vi "Husky Loop.vi"() -> ()   [LabVIEW 2011]
uses:
  clearpath_interface.lvlib
panel:
  in  "Set Velocity 2":bool
  in  "Translational Speed 2":dbl
  in  "Rotational Speed 2":dbl
  in  "Set Brake 2":bool
  in  "Continuous Vel 2":bool
  in  "Debug":bool
  in  "VISA resource name":refnum<visa-resource-name>
  out "Charge":dbl(slide) scale=0.0..100.0
  out "Left Speed (m/s)":dbl
  out "Right Speed (m/s)":dbl
  out "Capacity":i16
  out "Flags":u8 format="%b"
  out "Flags 2":u8 format="%x"
  in  "End Loop":bool
  in  "stop?":bool
  in  "Reset":bool
  in  "Max Accel":dbl
  in  "Set Max Accel":bool
  in  "Max Speed":dbl
  in  "Set Max Speed":bool
  in  "Set Velocity":bool
  in  "Translational Speed":dbl
  in  "Rotational Speed":dbl
  in  "Set Brake":bool
  in  "Continuous Vel":bool
  in  "Right Output":dbl
  in  "Left Output":dbl
  in  "Continuous Output":bool
  in  "Set Output":bool
  in  "P":dbl
  in  "I":dbl
  in  "D":dbl
  in  "FF":dbl
  in  "Stic":dbl
  in  "Int Lim":dbl
  in  "Set Controls":bool
  in  "Right Speed":dbl
  in  "Left Speed":dbl
  in  "Left Accel":dbl
  in  "Right Accel":dbl
  in  "Continuous Speeds":bool
  in  "Set Speeds":bool
  in  "Remote E-Stop":bool
  in  "Set Safety":bool
  in  "New Chassis Time (ms)":u32
  in  "Set Time":bool
  in  "New Chassis Name":string
  in  "Set Name":bool
  in  "FreqRawEncoder":u8
  in  "Update Raw Encoders":bool
  in  "Update Encoder":bool
  in  "FreqEncoder":u8
  in  "FreqPlatformRot":u8
  in  "Update Platform Rotation":bool
  in  "FreqMaxAccel":u8
  in  "Update Max Accel":bool
  in  "FreqMaxSpeed":u8
  in  "Update Max Speed":bool
  in  "FreqDifferentialOutput":u8
  in  "Update Differential Output":bool
  in  "FreqDifferentialControl":u8
  in  "Update Differential Control":bool
  in  "FreqDifferentialSpeed":u8
  in  "Update Differential Speed":bool
  in  "FreqSafetyStatus":u8
  in  "Update Safety Status":bool
  in  "FreqPowerSystem":u8
  in  "Update Power System":bool
  in  "FreqSystemStatus":u8
  in  "Update System Status":bool
  in  "FreqFirmwareInfo":u8
  in  "Update Firmware Info":bool
  in  "FreqPlatformName":u8
  in  "Update Platform Name":bool
  in  "FreqPlatformInfo":u8
  in  "Update Platform Info":bool
  # "Subscriptions"
  # "Communication Status"
  # "Platform Info (0x8001)"
  # "Differential Control (0x8201)"
  # "Platform Name (0x8002)"
  # "Differential Output (0x8202)"
  # "Firmware Info (0x8003)"
  # "Max Speed (0x8210)"
  # "System Status (0x8004)"
  # "Max Accel (0x8211)"
  # "Power System (0x8005)"
  # "Platform Rotation (0x8601)"
  # "Safety System Status (0x8010)"
  # "Encoders (0x8800)"
  # "Differential Speed (0x8200)"
  # "Raw Encoders (0x8801)"
  # "Set Velocity"
  # "Set Differential Speeds"
  # "Set Chassis Name/Time"
  # "Set Differential Controls"
  # "Set Differential Output"
  # "Set Max Speed/Accel"
  # "Set Safety System"
  # "Reset Processor"
  # "Control Test Panel\nClearpath Control Protocol cRIO Test Interface v1.0\nClearpath Robotics Inc., (c) 2010"
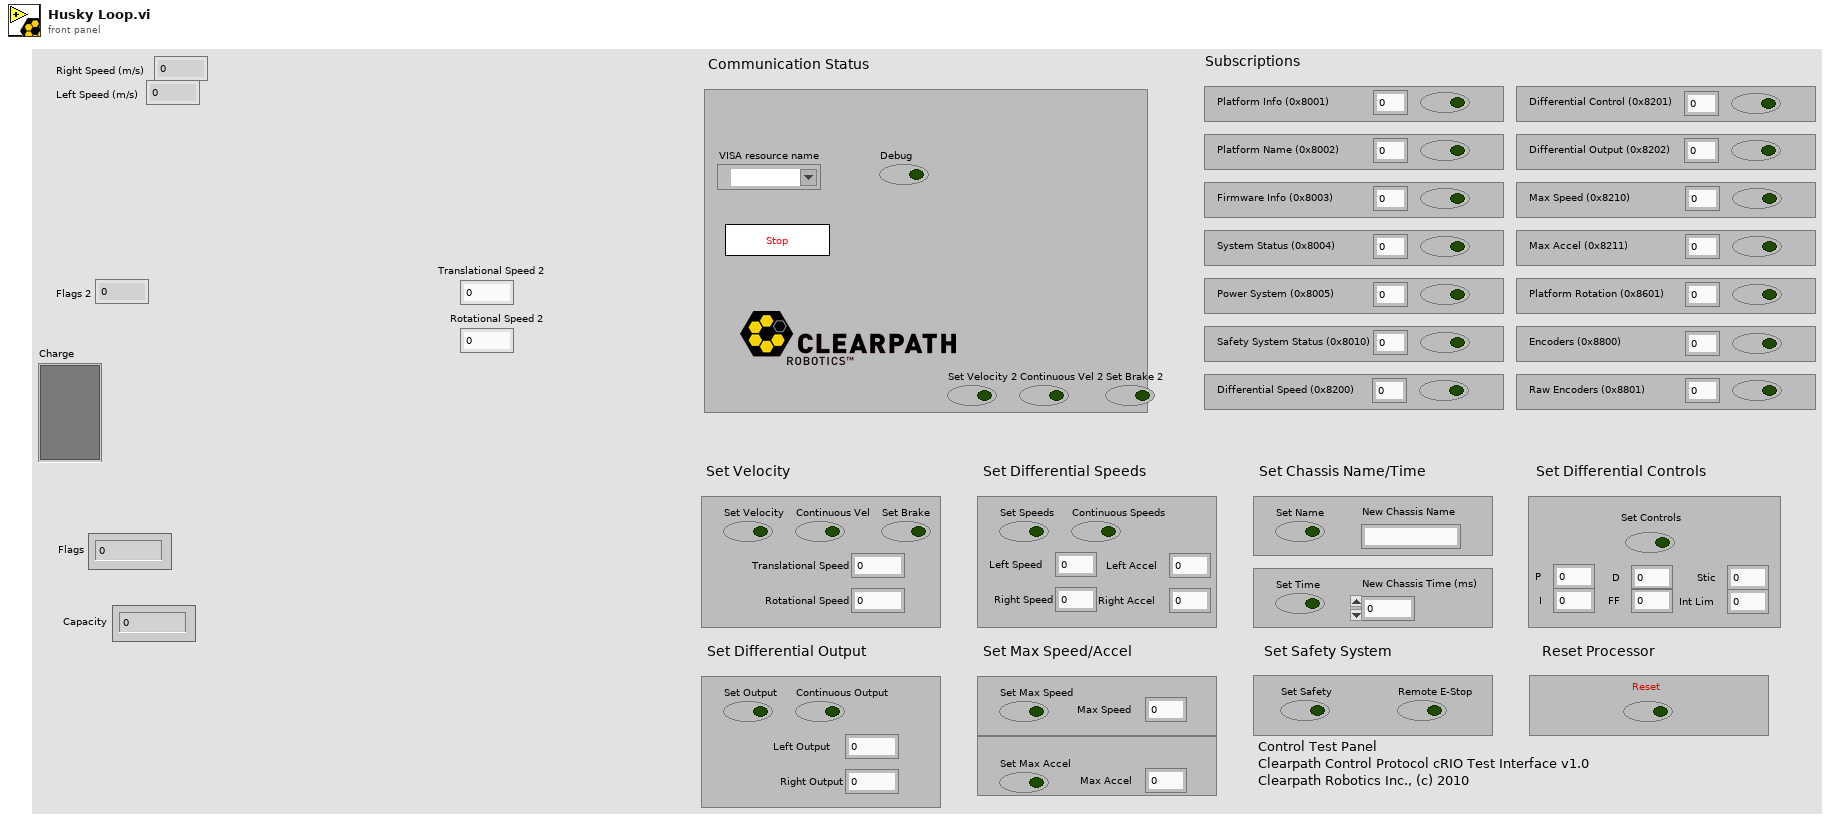
[diagram p1: front panel]
types:
  T1 = cluster{"P":dbl, "I":dbl, "D":dbl, "FF":dbl, "Stic":dbl, "Int Lim":dbl}
  T2 = cluster{"Xmit Queue":refnum<queue>, "Data Queue":refnum<queue>, "VISA resource name out":refnum<visa-resource-name>, "error out":errorcluster, "Message Data Cluster":cluster{"\nChar Idx":u8, "Num. Char Rem":u8, "Write Index":u8, "Read Index":u8, "Message Data Buffer":u8[][]}}
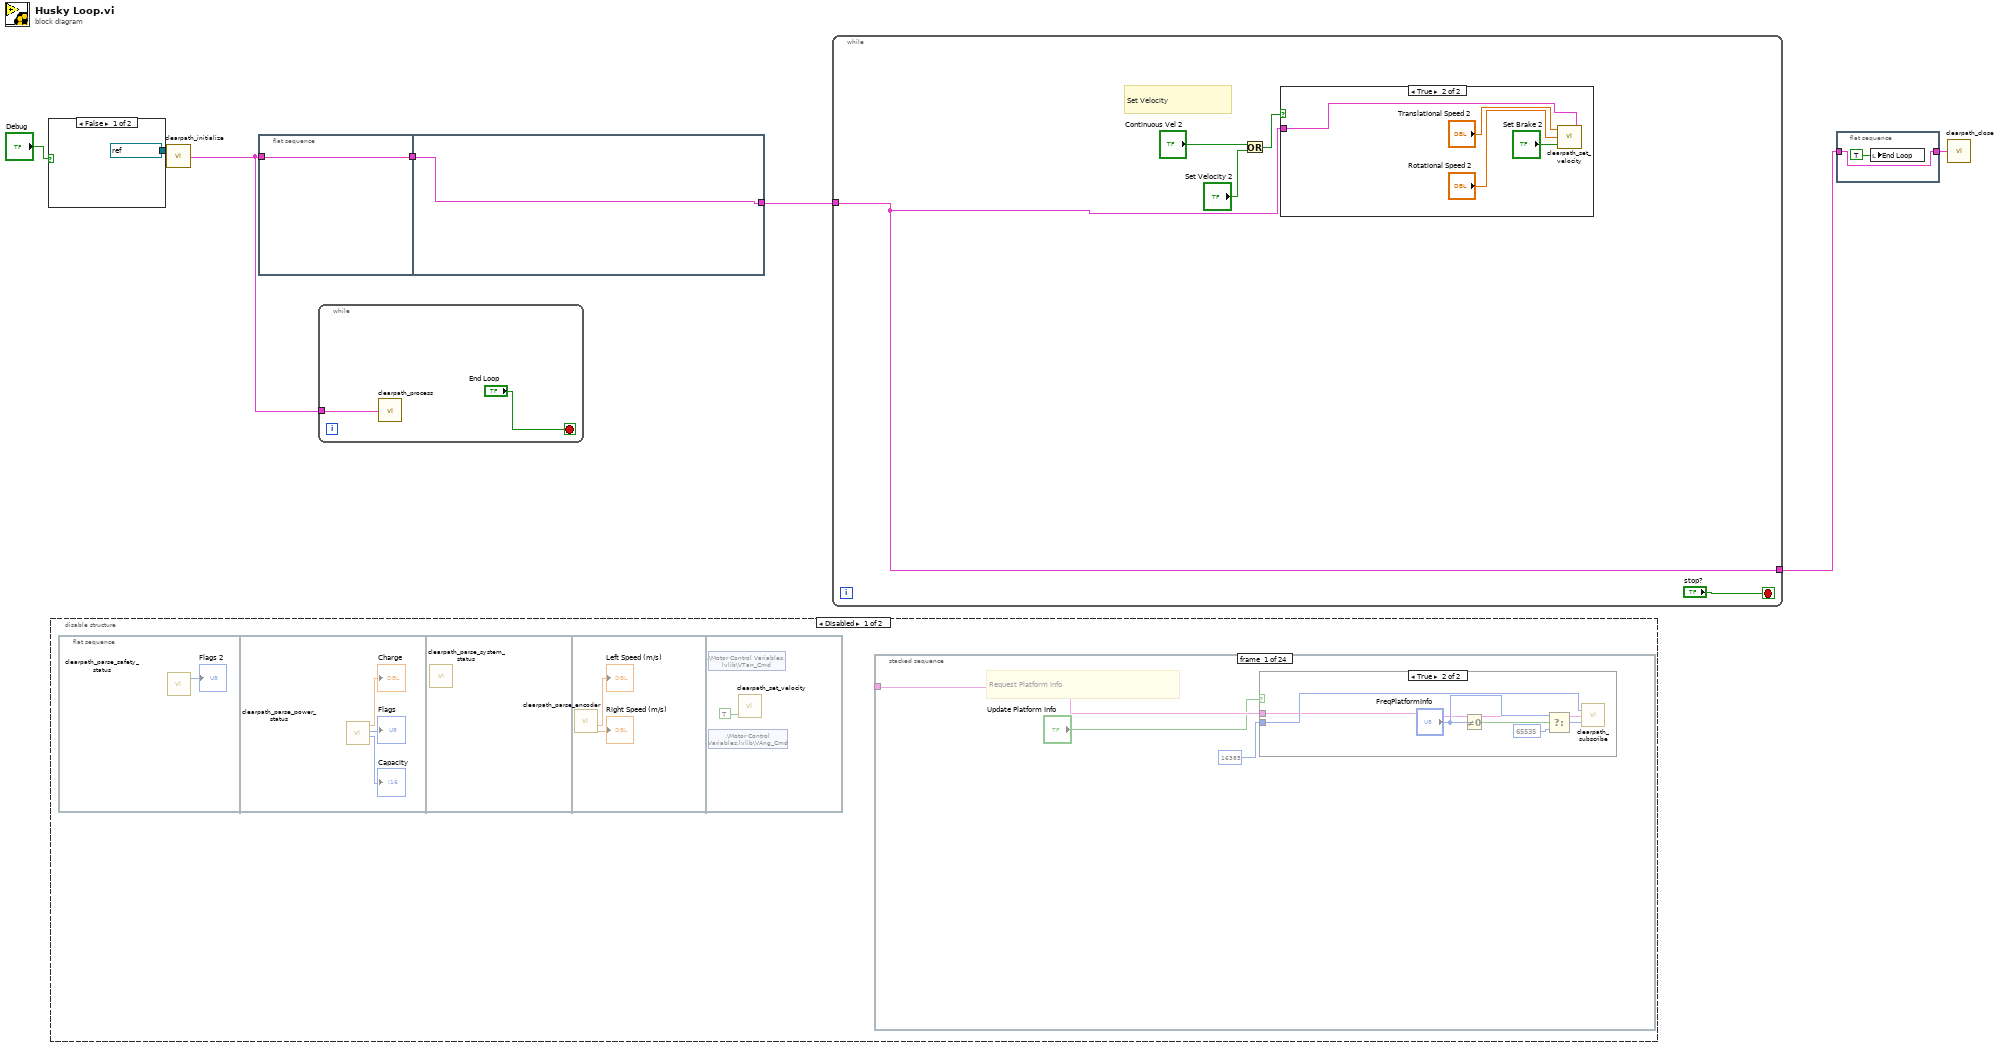
[diagram p0: block diagram]
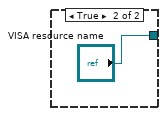
[diagram p3: hidden frame]
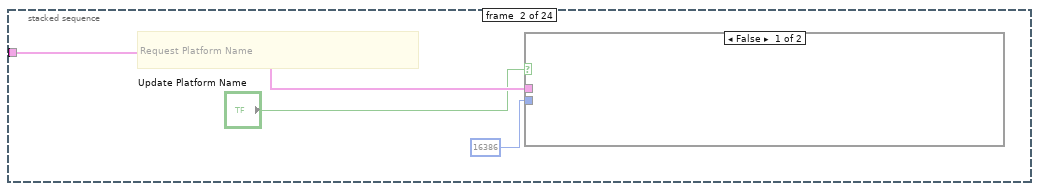
[diagram p5: hidden frame]
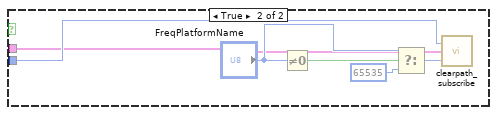
[diagram p6: hidden frame]
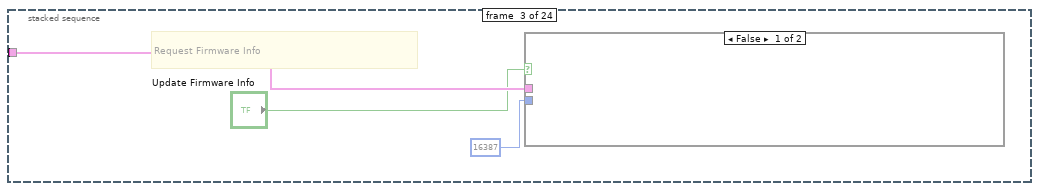
[diagram p7: hidden frame]
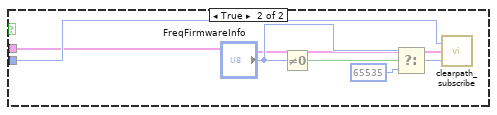
[diagram p8: hidden frame]
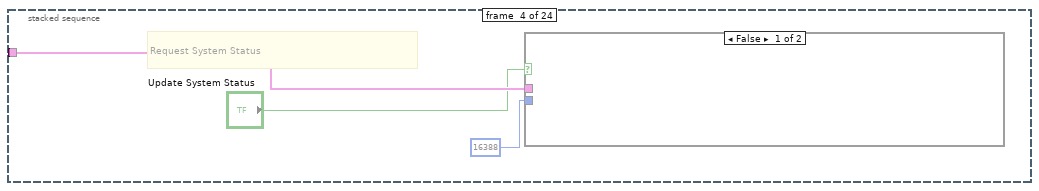
[diagram p9: hidden frame]
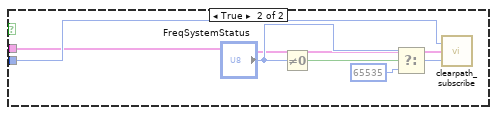
[diagram p10: hidden frame]
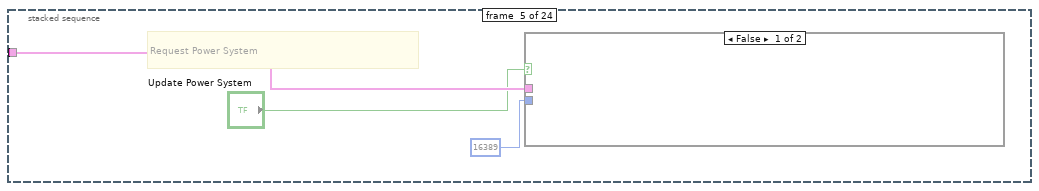
[diagram p11: hidden frame]
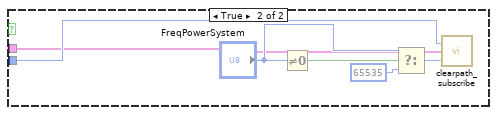
[diagram p12: hidden frame]
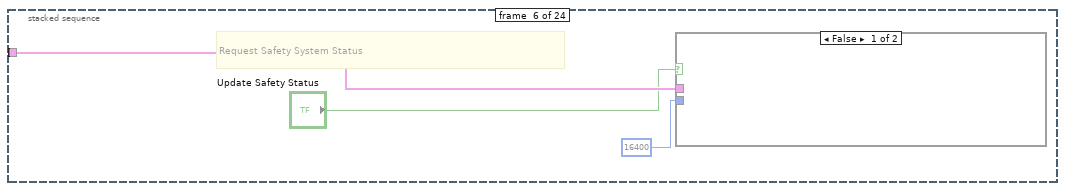
[diagram p13: hidden frame]
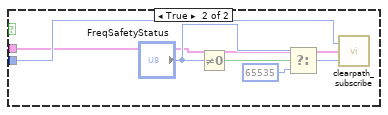
[diagram p14: hidden frame]
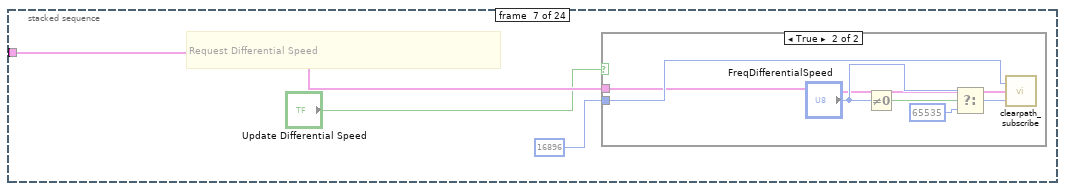
[diagram p15: hidden frame]
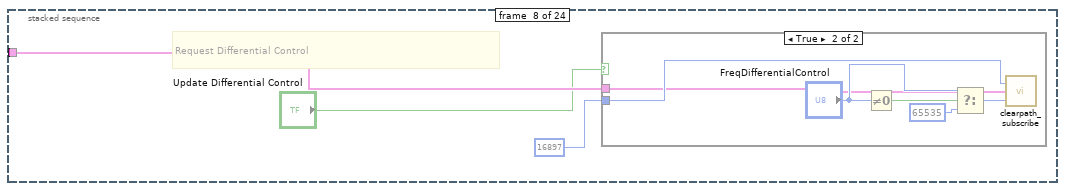
[diagram p17: hidden frame]
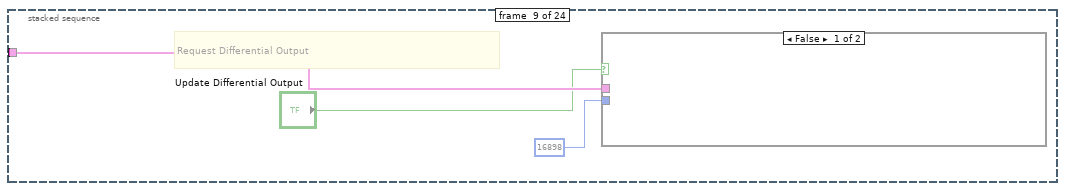
[diagram p19: hidden frame]
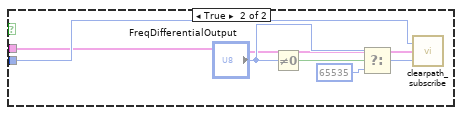
[diagram p20: hidden frame]
diagram:
  n1 = case shown="False" "Debug" {
    tunnel: [refnum<visa-resource-name> "COM15" ("VISA resource name") "VISA resource name"] -> w7
    frame False {
    }
    frame True {
    }
  }
  n2 = disable-structure shown="Disabled" {
    frame Disabled {
      n3 = flat-sequence {
        frame #0 {
          n4 = call "clearpath_parse_safety_status.vi"() -> ("Flags"=→"Flags 2":u8)  [unwired: 1 in, 1 out]
        }
        frame #1 {
          n5 = call "clearpath_parse_power_status.vi"() -> ("Capacity"=→"Capacity":i16, "Flags"=→"Flags":u8, "Charge"=→"Charge":dbl)  [unwired: 1 in, 1 out]
        }
        frame #2 {
          n6 = call "clearpath_parse_system_status.vi"() -> ()  [unwired: 1 in, 6 out]
        }
        frame #3 {
          n7 = call "clearpath_parse_encoder.vi"() -> ("Left Speed (m/s)"=→"Left Speed (m/s)":dbl, "Right Speed (m/s)"=→"Right Speed (m/s)":dbl)  [unwired: 1 in, 3 out]
        }
        frame #4 {
          n8 = shared-variable ".\\Motor Control Variables.lvlib\\VTan_Cmd"() -> ()  [unwired: 1 in, 2 out]
          n9 = shared-variable ".\\Motor Control Variables.lvlib\\VAng_Cmd"() -> ()  [unwired: 1 in, 2 out]
          n10 = call "clearpath_set_velocity.vi"("Zero Speeds"=TRUE) -> ()  [unwired: 3 in]
        }
      }
      n11 = stacked-sequence {
        tunnel: _ -> [w11 w21 w29 w38 w47 w56 w65 w74 w83 w92 w101 w111 w120 w129 w137 w141 w145 w150 w157 w168 w174 w181 w185 w189]
        frame #0 {
          # "Request Platform Info"
          n12 = case shown="True" "Update Platform Info" {
            tunnel: w11 -> [_ w13]
            tunnel: 16385 -> [_ w18]
            frame False {
            }
            frame True {
              n13 = Not Equal To 0?(x="FreqPlatformInfo") -> (x != 0?=w16:bool)
              n14 = Select(t="FreqPlatformInfo", s=w16, f=u16 65535) -> (s? t:f=w15:u16)
              n15 = call "clearpath_subscribe.vi"("ClearpathComm"=w13, "Frequency"=w15, "Message Type"=w18) -> ()
            }
          }
        }
        frame #1 {
          # "Request Platform Name"
          n16 = case shown="False" "Update Platform Name" {
            tunnel: w21 -> [_ w22]
            tunnel: 16386 -> [_ w27]
            frame False {
            }
            frame True {
              n17 = Not Equal To 0?(x="FreqPlatformName") -> (x != 0?=w25:bool)
              n18 = Select(t="FreqPlatformName", s=w25, f=u16 65535) -> (s? t:f=w24:u16)
              n19 = call "clearpath_subscribe.vi"("ClearpathComm"=w22, "Frequency"=w24, "Message Type"=w27) -> ()
            }
          }
        }
        frame #2 {
          # "Request Firmware Info"
          n20 = case shown="False" "Update Firmware Info" {
            tunnel: w29 -> [_ w31]
            tunnel: 16387 -> [_ w36]
            frame False {
            }
            frame True {
              n21 = Not Equal To 0?(x="FreqFirmwareInfo") -> (x != 0?=w34:bool)
              n22 = Select(t="FreqFirmwareInfo", s=w34, f=u16 65535) -> (s? t:f=w33:u16)
              n23 = call "clearpath_subscribe.vi"("ClearpathComm"=w31, "Frequency"=w33, "Message Type"=w36) -> ()
            }
          }
        }
        frame #3 {
          # "Request System Status"
          n24 = case shown="False" "Update System Status" {
            tunnel: w38 -> [_ w40]
            tunnel: 16388 -> [_ w45]
            frame False {
            }
            frame True {
              n25 = Not Equal To 0?(x="FreqSystemStatus") -> (x != 0?=w43:bool)
              n26 = Select(t="FreqSystemStatus", s=w43, f=u16 65535) -> (s? t:f=w42:u16)
              n27 = call "clearpath_subscribe.vi"("ClearpathComm"=w40, "Frequency"=w42, "Message Type"=w45) -> ()
            }
          }
        }
        frame #4 {
          # "Request Power System"
          n28 = case shown="False" "Update Power System" {
            tunnel: w47 -> [_ w49]
            tunnel: 16389 -> [_ w54]
            frame False {
            }
            frame True {
              n29 = Not Equal To 0?(x="FreqPowerSystem") -> (x != 0?=w52:bool)
              n30 = Select(t="FreqPowerSystem", s=w52, f=u16 65535) -> (s? t:f=w51:u16)
              n31 = call "clearpath_subscribe.vi"("ClearpathComm"=w49, "Frequency"=w51, "Message Type"=w54) -> ()
            }
          }
        }
        frame #5 {
          # "Request Safety System Status"
          n32 = case shown="False" "Update Safety Status" {
            tunnel: w56 -> [_ w58]
            tunnel: 16400 -> [_ w63]
            frame False {
            }
            frame True {
              n33 = Not Equal To 0?(x="FreqSafetyStatus") -> (x != 0?=w61:bool)
              n34 = Select(t="FreqSafetyStatus", s=w61, f=u16 65535) -> (s? t:f=w60:u16)
              n35 = call "clearpath_subscribe.vi"("ClearpathComm"=w58, "Frequency"=w60, "Message Type"=w63) -> ()
            }
          }
        }
        frame #6 {
          # "Request Differential Speed"
          n36 = case shown="True" "Update Differential Speed" {
            tunnel: w65 -> [_ w67]
            tunnel: 16896 -> [_ w72]
            frame False {
            }
            frame True {
              n37 = Not Equal To 0?(x="FreqDifferentialSpeed") -> (x != 0?=w70:bool)
              n38 = Select(t="FreqDifferentialSpeed", s=w70, f=u16 65535) -> (s? t:f=w69:u16)
              n39 = call "clearpath_subscribe.vi"("ClearpathComm"=w67, "Frequency"=w69, "Message Type"=w72) -> ()
            }
          }
        }
        frame #7 {
          # "Request Differential Control"
          n40 = case shown="True" "Update Differential Control" {
            tunnel: w74 -> [_ w76]
            tunnel: 16897 -> [_ w81]
            frame False {
            }
            frame True {
              n41 = Not Equal To 0?(x="FreqDifferentialControl") -> (x != 0?=w79:bool)
              n42 = Select(t="FreqDifferentialControl", s=w79, f=u16 65535) -> (s? t:f=w78:u16)
              n43 = call "clearpath_subscribe.vi"("ClearpathComm"=w76, "Frequency"=w78, "Message Type"=w81) -> ()
            }
          }
        }
        frame #8 {
          # "Request Differential Output"
          n44 = case shown="False" "Update Differential Output" {
            tunnel: w83 -> [_ w85]
            tunnel: 16898 -> [_ w90]
            frame False {
            }
            frame True {
              n45 = Not Equal To 0?(x="FreqDifferentialOutput") -> (x != 0?=w88:bool)
              n46 = Select(t="FreqDifferentialOutput", s=w88, f=u16 65535) -> (s? t:f=w87:u16)
              n47 = call "clearpath_subscribe.vi"("ClearpathComm"=w85, "Frequency"=w87, "Message Type"=w90) -> ()
            }
          }
        }
        frame #9 {
          # "Request Max Speed"
          n48 = case shown="False" "Update Max Speed" {
            tunnel: w92 -> [_ w94]
            tunnel: 16912 -> [_ w99]
            frame False {
            }
            frame True {
              n49 = Not Equal To 0?(x="FreqMaxSpeed") -> (x != 0?=w97:bool)
              n50 = Select(t="FreqMaxSpeed", s=w97, f=u16 65535) -> (s? t:f=w96:u16)
              n51 = call "clearpath_subscribe.vi"("ClearpathComm"=w94, "Frequency"=w96, "Message Type"=w99) -> ()
            }
          }
        }
        frame #10 {
          # "Request Max Accel"
          n52 = case shown="False" "Update Max Accel" {
            tunnel: w101 -> [_ w103]
            tunnel: 16913 -> [_ w108]
            frame False {
            }
            frame True {
              n53 = Not Equal To 0?(x="FreqMaxAccel") -> (x != 0?=w106:bool)
              n54 = Select(t="FreqMaxAccel", s=w106, f=u16 65535) -> (s? t:f=w105:u16)
              n55 = call "clearpath_subscribe.vi"("ClearpathComm"=w103, "Frequency"=w105, "Message Type"=w108) -> ()
            }
          }
        }
        frame #11 {
          # "Request Platform Rotation"
          n56 = case shown="False" "Update Platform Rotation" {
            tunnel: w111 -> [_ w112]
            tunnel: 17921 -> [_ w117]
            frame False {
            }
            frame True {
              n57 = Not Equal To 0?(x="FreqPlatformRot") -> (x != 0?=w115:bool)
              n58 = Select(t="FreqPlatformRot", s=w115, f=u16 65535) -> (s? t:f=w114:u16)
              n59 = call "clearpath_subscribe.vi"("ClearpathComm"=w112, "Frequency"=w114, "Message Type"=w117) -> ()
            }
          }
        }
        frame #12 {
          # "Request Encoders"
          n60 = case shown="False" "Update Encoder" {
            tunnel: w120 -> [_ w121]
            tunnel: 18432 -> [_ w126]
            frame False {
            }
            frame True {
              n61 = Not Equal To 0?(x="FreqEncoder") -> (x != 0?=w123:bool)
              n62 = Select(t="FreqEncoder", s=w123, f=u16 65535) -> (s? t:f=w122:u16)
              n63 = call "clearpath_subscribe.vi"("ClearpathComm"=w121, "Frequency"=w122, "Message Type"=w126) -> ()
            }
          }
        }
        frame #13 {
          # "Request Raw Encoders"
          n64 = case shown="False" "Update Raw Encoders" {
            tunnel: w129 -> [_ w130]
            tunnel: 18433 -> [_ w135]
            frame False {
            }
            frame True {
              n65 = Not Equal To 0?(x="FreqRawEncoder") -> (x != 0?=w133:bool)
              n66 = Select(t="FreqRawEncoder", s=w133, f=u16 65535) -> (s? t:f=w132:u16)
              n67 = call "clearpath_subscribe.vi"("ClearpathComm"=w130, "Frequency"=w132, "Message Type"=w135) -> ()
            }
          }
        }
        frame #14 {
          # "Set Platform Name"
          n68 = case shown="False" "Set Name" {
            tunnel: w137 -> [_ w138]
            frame False {
            }
            frame True {
              n69 = call "clearpath_set_platform_name.vi"("ClearpathComm"=w138, "New Name"="New Chassis Name") -> ()
            }
          }
        }
        frame #15 {
          # "Set Platform Time"
          n70 = case shown="False" "Set Time" {
            tunnel: w141 -> [_ w142]
            frame False {
            }
            frame True {
              n71 = call "clearpath_set_platform_time.vi"("ClearpathComm"=w142, "New Time"="New Chassis Time (ms)") -> ()
            }
          }
        }
        frame #16 {
          # "Set Safety System"
          n72 = case shown="False" "Set Safety" {
            tunnel: w145 -> [_ _]
            frame False {
            }
            frame True {
              n73 = call "clearpath_set_safety_system.vi"("Set Stop Flag"="Remote E-Stop") -> ()  [unwired: 1 in]
            }
          }
        }
        frame #17 {
          # "Set Differential Speeds"
          n74 = Or(x="Continuous Speeds", y="Set Speeds") -> (x .or. y?=w148:bool)
          n75 = case shown="False" w148 {
            tunnel: w150 -> [_ w151]
            frame False {
            }
            frame True {
              n76 = call "clearpath_set_differential_speeds.vi"("ClearpathComm"=w151, "Right Accel"="Right Accel", "Left Accel"="Left Accel", "Right Speed"="Right Speed", "Left Speed"="Left Speed") -> ()
            }
          }
        }
        frame #18 {
          # "Set Differential Controls"
          n77 = case shown="False" "Set Controls" {
            tunnel: w157 -> [_ _]
            frame False {
            }
            frame True {
              n78 = Bundle("P"="P", "I"="I", "D"="D", "FF"="FF", "Stic"="Stic", "Int Lim"="Int Lim") -> (w158:T1)  [unwired: 1 in]
              n79 = call "clearpath_set_differential_controls.vi"("Controls Cluster"=w158) -> ()  [unwired: 1 in]
            }
          }
        }
        frame #19 {
          # "Set Differential Output"
          n80 = Or(x="Continuous Output", y="Set Output") -> (x .or. y?=w166:bool)
          n81 = case shown="True" w166 {
            tunnel: w168 -> [_ w169]
            frame False {
            }
            frame True {
              n82 = call "clearpath_set_differential_output.vi"("ClearpathComm"=w169, "Right Output"="Right Output", "Left Output"="Left Output") -> ()
            }
          }
        }
        frame #20 {
          # "Set Velocity"
          n83 = Or(x="Continuous Vel", y="Set Velocity") -> (x .or. y?=w173:bool)
          n84 = case shown="True" w173 {
            tunnel: w174 -> [_ w176]
            frame False {
            }
            frame True {
              n85 = call "clearpath_set_velocity.vi"("ClearpathComm"=w176, "Zero Speeds"="Set Brake", "Rotational Speed"="Rotational Speed", "Translational Speed"="Translational Speed") -> ()
            }
          }
        }
        frame #21 {
          # "Set Max Speed"
          n86 = case shown="True" "Set Max Speed" {
            tunnel: w181 -> [_ w182]
            frame False {
            }
            frame True {
              n87 = call "clearpath_set_max_speed.vi"("ClearpathComm"=w182, "Max Speed"="Max Speed") -> ()
            }
          }
        }
        frame #22 {
          # "Set Max Accel"
          n88 = case shown="True" "Set Max Accel" {
            tunnel: w185 -> [_ w186]
            frame False {
            }
            frame True {
              n89 = call "clearpath_set_max_accel.vi"("ClearpathComm"=w186, "Max Accel"="Max Accel") -> ()
            }
          }
        }
        frame #23 {
          # "Reset Processor"
          n90 = case shown="True" "Reset" {
            tunnel: w189 -> [_ _]
            frame False {
            }
            frame True {
            }
          }
        }
      }
    }
    frame Enabled {
    }
  }
  n91 = call "clearpath_initialize.vi"("VISA resource name"=w7) -> ("ClearpathComm"=w6:T2)  [unwired: 1 in]
  n92 = flat-sequence {
    tunnel: w6 -> [w197]
    tunnel: [w197] -> w5
    tunnel: w5 -> [w198]
    tunnel: [w198] -> w4
    frame #0 {
    }
    frame #1 {
    }
  }
  n93 = while {
    tunnel: w6 -> [w200]
    stop <- "End Loop" stop-if-true
    n94 = call "clearpath_process.vi"("ClearpathComm"=w200) -> ()
  }
  n95 = while {
    tunnel: w4 -> [w201]
    tunnel: [w201] -> w2
    stop <- "stop?" stop-if-true
    # "Set Velocity"
    n96 = Or(x="Continuous Vel 2", y="Set Velocity 2") -> (x .or. y?=w203:bool)
    n97 = case shown="True" w203 {
      tunnel: w201 -> [_ w206]
      frame False {
      }
      frame True {
        n98 = call "clearpath_set_velocity.vi"("ClearpathComm"=w206, "Zero Speeds"="Set Brake 2", "Rotational Speed"="Rotational Speed 2", "Translational Speed"="Translational Speed 2") -> ()
      }
    }
  }
  n99 = flat-sequence {
    tunnel: [w210] -> w3
    tunnel: w2 -> [w210]
    frame #0 {
      n100 = local write "End Loop"(TRUE ("End Loop")) -> ()
    }
  }
  n101 = call "clearpath_close.vi"("ClearpathComm"=w3) -> ()
